vi "Get Type of a Hand.vi"(0 "Cards in a hand":string[](array[string]), 1 "F:J is Normal Card | T:J is Joker Card (F)":bool) -> (2 "Type":T1=enum."Five of a kind")   [LabVIEW 2020, in "AoC 2023.lvlib"]
uses:
  AoC 2023.lvlib
  Type of a Hand.ctl
  <vilib>/Utility/miscctls.llb/LVMapReplaceAction.ctl
  4959147c-7566-49fe-a844-b16dfe421289.vi
  a484e149-5bf0-46bd-874a-32713ee95b42.vi
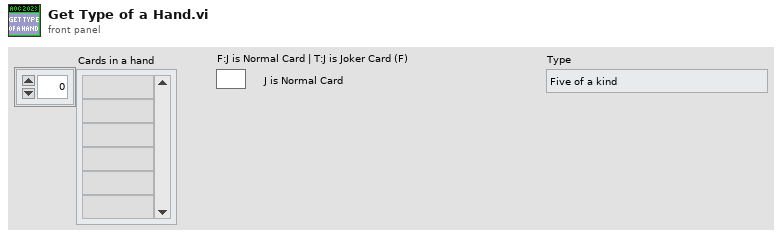
[diagram p1: front panel]
types:
  T1 = typedef "AoC 2023.lvlib/Type of a Hand.ctl" = enum16{"High card", "One pair", "Two pair", "Three of a kind", "Full house", "Four of a kind", "Five of a kind", "Unknown"}
  T2 = typedef "LVMapReplaceAction.ctl" = enum32{"Modify Entry only if found", "Add or Modify Entry", "Delete Entry"}
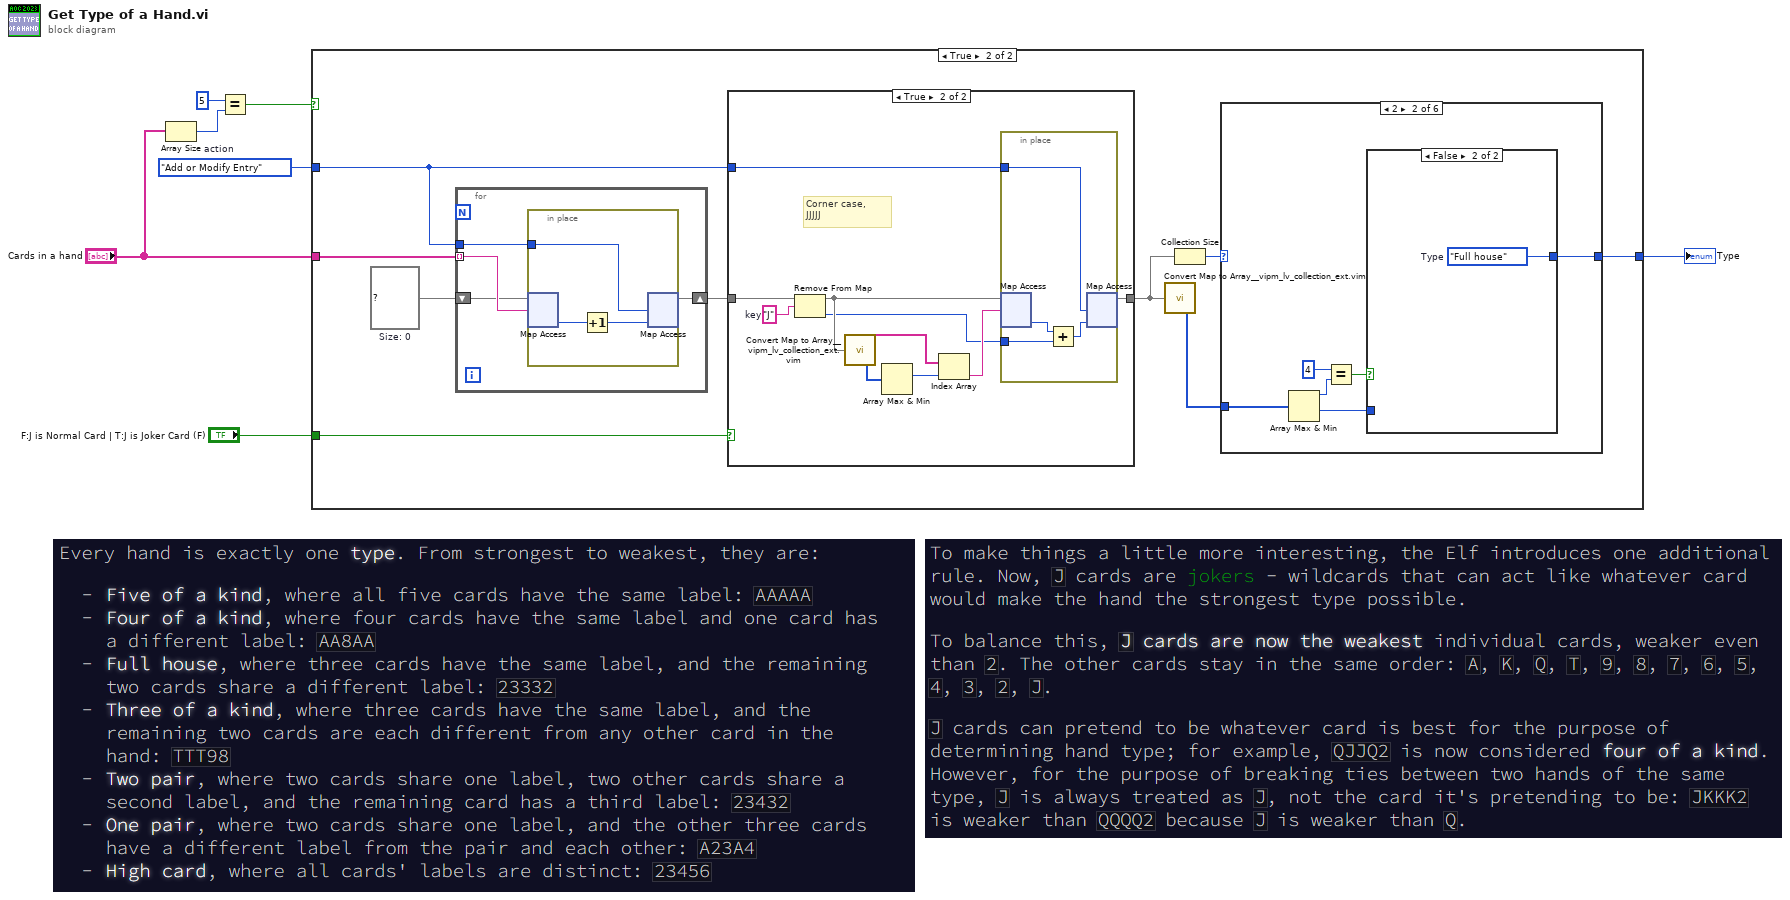
[diagram p0: block diagram]
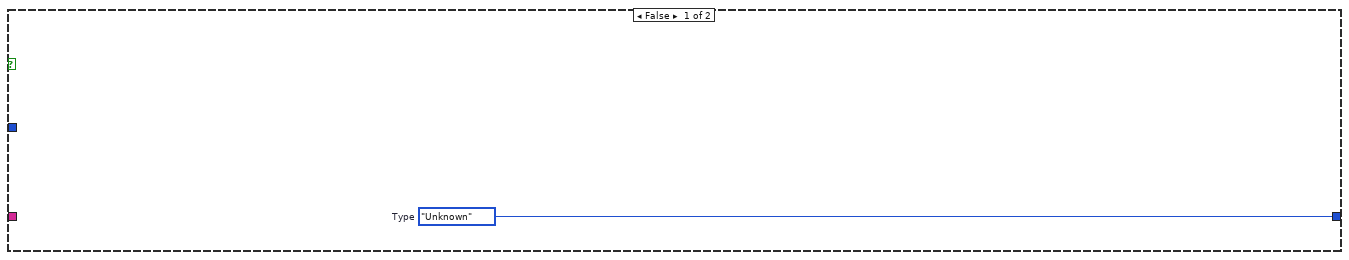
[diagram p2: hidden frame]
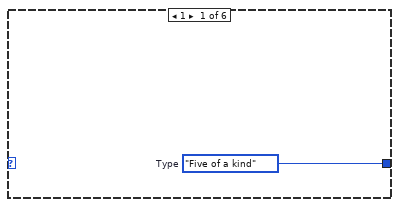
[diagram p4: hidden frame]
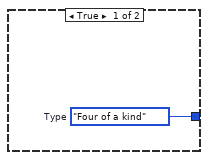
[diagram p5: hidden frame]
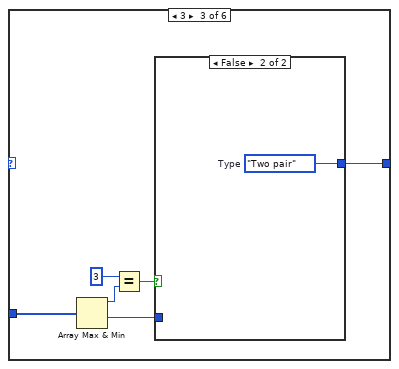
[diagram p6: hidden frame]
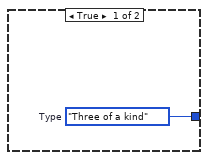
[diagram p7: hidden frame]
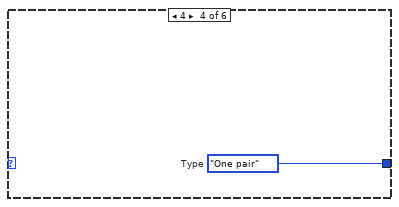
[diagram p8: hidden frame]
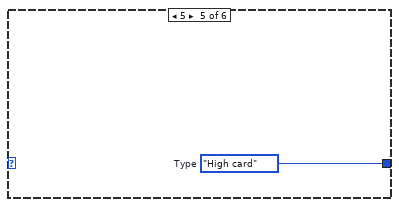
[diagram p9: hidden frame]
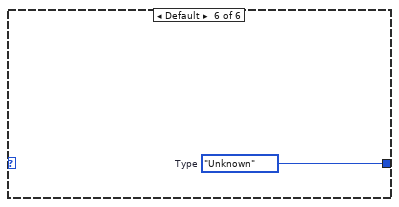
[diagram p10: hidden frame]
diagram:
  w1 = LVMapReplaceAction."Add or Modify Entry"  # action
  n1 = Array Size(array="Cards in a hand") -> (size(s)=w7:i32)
  n2 = Equal?(x=5, y=w7) -> (x = y?=w4:bool)
  n3 = case shown="True" w4 {
    tunnel: [w8 w16] -> w5
    tunnel: "Cards in a hand" -> [_ w15]
    tunnel: "F:J is Normal Card | T:J is Joker Card (F)" -> [_ w10]
    tunnel: w1 -> [_ w9]
    frame False {
      w8 = Type_of_a_Hand."Unknown"  # Type
    }
    frame True {
      w14 = map{string, i32} {}  # Size: 0
      n4 = for {
        tunnel: w15 -> [w36] mode=indexing
        shift-right: [w35] -> w13
        shift-left: w14 -> [w34]
        tunnel: w9 -> [w33]
        n5 = in-place {
          in-place-border: w33 -> [w37]
          n6 = in-place-map #1(w34, w36) -> (w39:i32)  [unwired: 1 in, 1 out]
          n7 = Increment(x=w39) -> (x+1=w38:i32)
          n8 = in-place-map #1(w38, w37) -> (w35:map{string, i32})  [unwired: 2 out]
        }
      }
      n9 = case shown="True" w10 {
        tunnel: w13 -> [w18 w28]
        tunnel: [w18 w22] -> w12
        tunnel: w9 -> [_ w19]
        frame False {
        }
        frame True {
          w27 = "J"  # key
          # "Corner case,\nJJJJJ"
          n10 = Remove From Map(10:w27, 11:w28) -> (1:w23:i32, 3:w25:map{string, i32})  [unwired: 1 out]
          n11 = call "Convert Map to Array__vipm_lv_collection_ext.vim"("map"=w25) -> ("keys"=w26:string[], "values"=w21:i32[])  [unwired: 12 in, 1 out]
          n12 = Array Max & Min(array=w21) -> (max index (indices)=w20:i32)  [unwired: 3 out]
          n13 = Index Array(array=w26, index=w20) -> (element=w24:string)
          n14 = in-place {
            in-place-border: w23 -> [w31]
            in-place-border: w19 -> [w29]
            n15 = in-place-map #2(w25, w24) -> (w32:i32)  [unwired: 1 in, 1 out]
            n16 = Add(x=w32, y=w31) -> (x+y=w30:i32)
            n17 = in-place-map #2(w30, w29) -> (w22:map{string, i32})  [unwired: 2 out]
          }
        }
      }
      n18 = call "Convert Map to Array__vipm_lv_collection_ext.vim"("map"=w12) -> ("values"=w11:i32[])  [unwired: 12 in, 2 out]
      n19 = Collection Size(1:w12) -> (0:w17:i32)
      n20 = case shown="2" w17 {
        tunnel: [w40 w46 w54 w57 w58 w59] -> w16
        tunnel: w11 -> [_ w41 w49 _ _ _]
        frame 1 {
          w40 = Type_of_a_Hand."Five of a kind"  # Type
        }
        frame 2 {
          n21 = Array Max & Min(array=w41) -> (max value=w45:i32, min value=w42:i32)  [unwired: 2 out]
          n22 = Equal?(x=4, y=w45) -> (x = y?=w43:bool)
          n23 = case shown="False" w43 {
            tunnel: [w47 w48] -> w46
            tunnel: w42 -> [_ _]
            frame True {
              w47 = Type_of_a_Hand."Four of a kind"  # Type
            }
            frame False {
              w48 = Type_of_a_Hand."Full house"  # Type
            }
          }
        }
        frame 3 {
          n24 = Array Max & Min(array=w49) -> (max value=w53:i32, min value=w50:i32)  [unwired: 2 out]
          n25 = Equal?(x=3, y=w53) -> (x = y?=w51:bool)
          n26 = case shown="False" w51 {
            tunnel: [w55 w56] -> w54
            tunnel: w50 -> [_ _]
            frame True {
              w55 = Type_of_a_Hand."Three of a kind"  # Type
            }
            frame False {
              w56 = Type_of_a_Hand."Two pair"  # Type
            }
          }
        }
        frame 4 {
          w57 = Type_of_a_Hand."One pair"  # Type
        }
        frame 5 {
          w58 = Type_of_a_Hand."High card"  # Type
        }
        frame Default {
          w59 = Type_of_a_Hand."Unknown"  # Type
        }
      }
    }
  }
  "Type" <- w5
